vi "SJ_Get_Signal_Phase.vi"(8 "No of Analogue Samples":i32=600, 9 "Number of Cycles":i32=1, 10 "Actual Sampling Frequency":dbl=12000.0, 11 "Signal":dbl[](array[numeric])) -> (3 "Phase Angle _deg_":dbl)   [LabVIEW 2011]
uses:
  <vilib>/Analysis/2dsp.llb/1D Cross Correlation (DBL).vi
  <vilib>/Analysis/NI_AALBase.lvlib
  <vilib>/Analysis/NI_AALPro.lvlib
  <vilib>/Analysis/NI_AAL_SigProc.lvlib
panel:
  out "Waveform Graph":dbl[](graph)
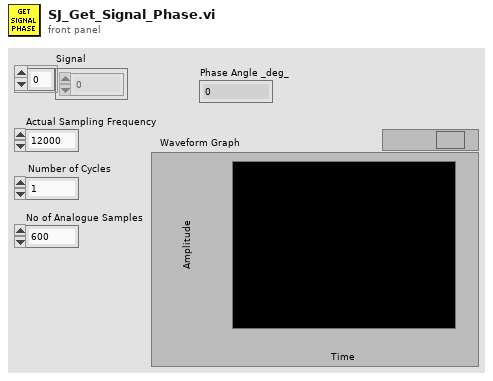
[diagram p1: front panel]
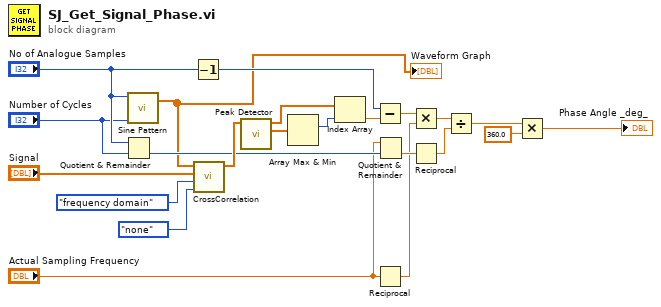
[diagram p0: block diagram]
diagram:
  n1 = Quotient & Remainder(x="No of Analogue Samples", y="Number of Cycles") -> (floor(x/y)=w16:i32)  [unwired: 1 out]
  n2 = call <vilib>:"Sine Pattern.vi"("cycles"="Number of Cycles", "samples"="No of Analogue Samples") -> ("Sinusoidal Pattern"=w1:dbl[])  [unwired: 2 in, 1 out]
  "Waveform Graph" <- w1
  n3 = Decrement(x="No of Analogue Samples") -> (x-1=w6:i32)
  n4 = call-poly <vilib>:"CrossCorrelation.vi"("normalization"=enum32{"none", "unbiased", "biased"}."none", "algorithm"=enum32{"direct", "frequency domain"}."frequency domain", "Y"="Signal", "X"=w1) -> ("Rxy"=w21:dbl[])  [unwired: 6 in, 1 out]
  n5 = call <vilib>:"Peak Detector.vi"("X"=w21) -> ("Amplitudes"=w20:dbl[], "Locations"=w19:dbl[])  [unwired: 6 in, 3 out]
  n6 = Array Max & Min(array=w20) -> (max index (indices)=w18:i32)  [unwired: 3 out]
  n7 = Index Array(array=w19, index=w18) -> (element=w5:dbl)
  n8 = Subtract(x=w6, y=w5) -> (x-y=w13:dbl)
  n9 = Reciprocal(x="Actual Sampling Frequency") -> (1/x=w12:dbl)
  n10 = Quotient & Remainder(x="Actual Sampling Frequency", y=w16) -> (floor(x/y)=w14:dbl)  [unwired: 1 out]
  n11 = Multiply(x=w13, y=w12) -> (x*y=w10:dbl)
  n12 = Reciprocal(x=w14) -> (1/x=w11:dbl)
  n13 = Divide(x=w10, y=w11) -> (x/y=w9:dbl)
  n14 = Multiply(x=w9, y=360.0) -> (x*y=→"Phase Angle _deg_":dbl)
